vi "Initialize Values.vi"(8 "error in (no error)":errorcluster, 11 "Scale Calibration in":refnum<class "Scale Calibration.lvclass">) -> (0 "error out":errorcluster, 3 "Scale Calibration out":refnum<class "Scale Calibration.lvclass">)   [LabVIEW 2014, in "SeqLoop.lvlib" / "STEP Classes.lvlib" / "Scale Calibration.lvclass"]
uses:
  Scale Calibration.lvclass
  Scale Calibration.lvclass/Scale Calibration.ctl
  STEP/STEP.lvclass
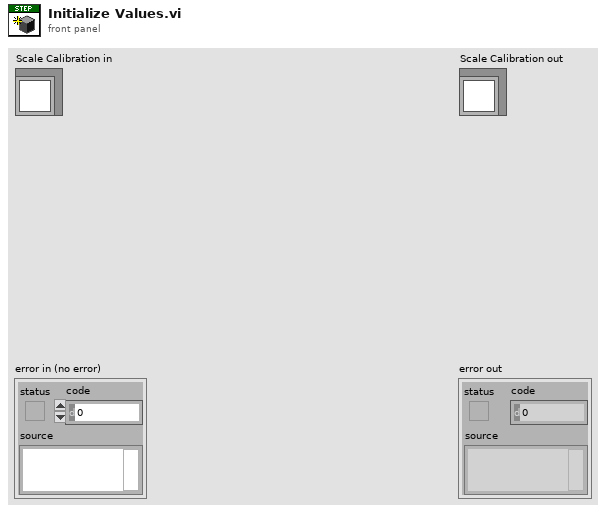
[diagram p1: front panel]
types:
  T1 = cluster{"HWSync 1":bool, "HWSync 2":bool, "HWSync 3":bool, "HWSync 4":bool, "HWSync 5":bool}
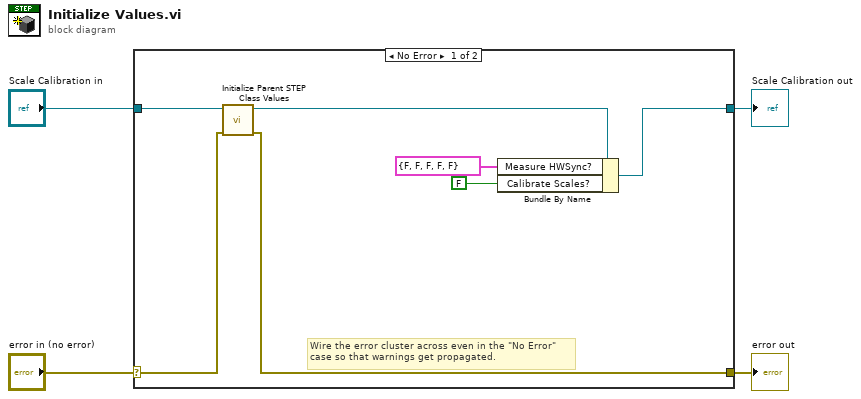
[diagram p0: block diagram]
diagram:
  n1 = case shown="No Error" "error in (no error)" {
    selector: "error in (no error)" -> [w10 w13]
    tunnel: [w9 w13] -> w3
    tunnel: [w7 w12] -> w1
    tunnel: "Scale Calibration in" -> [w11 w12]
    frame No Error {
      # "Wire the error cluster across even in the \"No Error\"\ncase so that warnings get propagated."
      n2 = call "Initialize Parent STEP Class Values.vi"("error in (no error)"=w10, "STEP in"=w11) -> ("error out"=w9:errorcluster, "STEP out"=w8:refnum<class "Scale Calibration.lvclass">)  [unwired: 8 in]
      n3 = Bundle By Name(cluster=w8, "Measure HWSync?"=T1 {"HWSync 1"=FALSE, "HWSync 2"=FALSE, "HWSync 3"=FALSE, "HWSync 4"=FALSE, "HWSync 5"=FALSE}, "Calibrate Scales?"=FALSE) -> (w7:refnum<class "Scale Calibration.lvclass">)
    }
    frame Error {
    }
  }
  "error out" <- w3
  "Scale Calibration out" <- w1
